vi "TestFastLocalizeCPU.vi"() -> ()   [LabVIEW 2011]
panel:
  out "debug image":T1(plugin-control)
  out "Image":T1(plugin-control)
  out "median":sgl
  out "xcorpos":cluster{"XCor X":sgl, "XCor Y":sgl}
  out "COM":cluster{"comX":sgl, "comY":sgl}
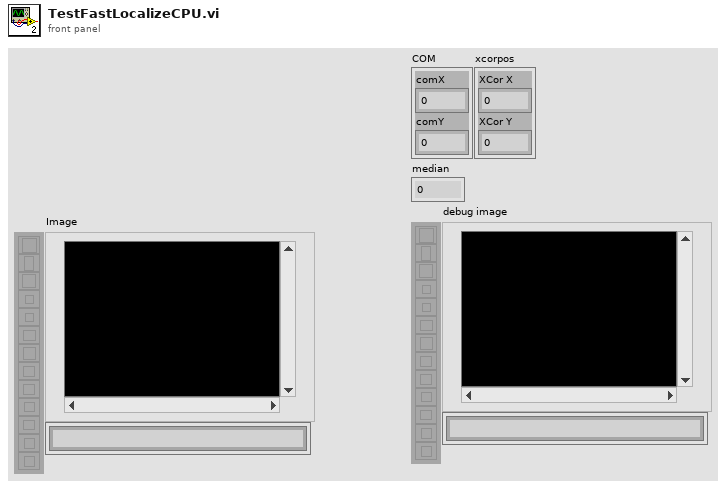
[diagram p1: front panel]
types:
  T1 = typedef "IMAQ Image.ctl" = refnum<image>
  T2 = typedef "Image Type" = u32
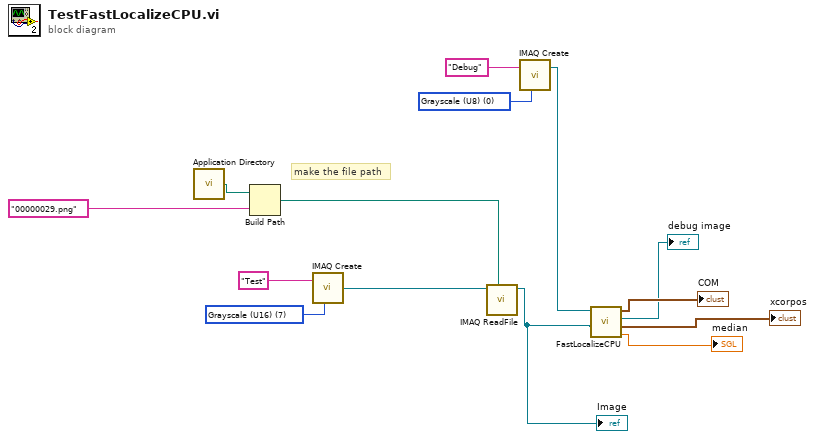
[diagram p0: block diagram]
diagram:
  w3 = T2 0 items=["Grayscale (U8)", "Grayscale (I16)", "Grayscale (SGL)", "Complex (CSG)", "RGB (U32)", "HSL (U32)", "RGB (U64)", "Grayscale (U16)"] ("Image Type")
  w5 = T2 7 items=["Grayscale (U8)", "Grayscale (I16)", "Grayscale (SGL)", "Complex (CSG)", "RGB (U32)", "HSL (U32)", "RGB (U64)", "Grayscale (U16)"] ("Image Type")
  # "make the file path"
  n1 = call <vilib>:"Application Directory.vi"() -> ("Application Directory"=w12:path)
  n2 = Build Path(base path=w12, name or relative path="00000029.png") -> (appended path=w10:path)
  n3 = call "IMAQ Create"("Image Name"="Test" ("String"), "Image Type"=w5) -> ("New Image"=w13:T1)  [unwired: 3 in, 1 out]
  n4 = call "IMAQ ReadFile"("File Path"=w10, "Image"=w13) -> ("Image Out"=w9:T1)  [unwired: 5 in, 4 out]
  "Image" <- w9
  n5 = call "IMAQ Create"("Image Name"="Debug" ("String"), "Image Type"=w3) -> ("New Image"=w2:T1)  [unwired: 3 in, 1 out]
  n6 = call "FastLocalizeCPU.vi"("Image"=w9, "debug image"=w2) -> ("median"=→"median":sgl, "xcorpos"=→"xcorpos":cluster{"XCor X":sgl, "XCor Y":sgl}, "debug image"=→"debug image":T1, "COM"=→"COM":cluster{"comX":sgl, "comY":sgl})  [unwired: 2 in]
